vi "Delete Thing Shadow.vi"(8 "error in (no error)":errorcluster, 11 "Thing Shadow":refnum<class "Thing Shadow.lvclass">) -> (0 "error out":errorcluster)   [LabVIEW 2015, in "NI_AWS_IoT.lvlib" / "Thing Shadow.lvclass"]
uses:
  Thing Shadow.lvclass
  Core/HTTP Request/Request Options.ctl
  Core/HTTP Request/Name Value Pair.ctl
  Core/HTTP Request/Region handling.ctl
  Core/HTTP Request/URL formatting.ctl
  Thing Shadow.lvclass/Thing Shadow.ctl
  Read Thing Name.vi
  Core/HTTP Request/HTTP Request.lvclass
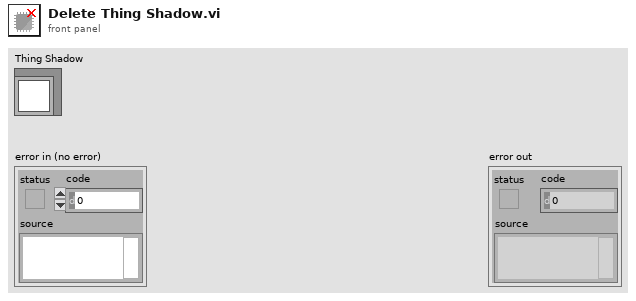
[diagram p1: front panel]
types:
  T1 = typedef "NI_AWS_Core.lvlib/HTTP Request.lvclass/Name Value Pair.ctl" = cluster{"name":string, "value":string}
  T2 = typedef "NI_AWS_Core.lvlib/HTTP Request.lvclass/Request Options.ctl" = cluster{"request headers":T1[], "request parameters":T1[], "request body":string, "region handling":T3, "URL formatting":T4}
  T3 = typedef "NI_AWS_Core.lvlib/HTTP Request.lvclass/Region handling.ctl" = enum16{"use region everywhere", "use region (authentication only)", "use region (URL only)", "ignore region everwhere"}
  T4 = typedef "NI_AWS_Core.lvlib/HTTP Request.lvclass/URL formatting.ctl" = enum16{"region-", "region."}
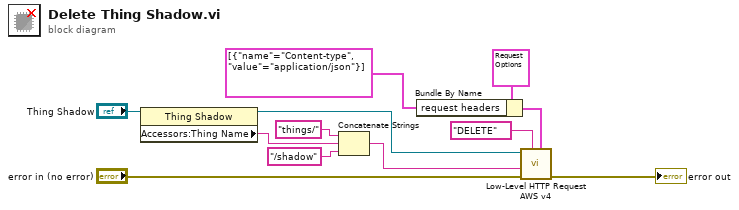
[diagram p0: block diagram]
diagram:
  n1 = property class="Thing Shadow"(reference="Thing Shadow") -> (reference out=w3:refnum<class "Thing Shadow.lvclass">, "Accessors:Thing Name"=w2:string)  [unwired: 1 in, 1 out]
  n2 = Concatenate Strings("things/" ("string"), w2, "/shadow" ("string")) -> (w7:string)
  n3 = Bundle By Name(cluster=T2 {"request headers"=[], "request parameters"=[], "request body"="", "region handling"=enum."use region everywhere", "URL formatting"=enum."region."} ("Request Options"), "request headers"=T1[] [{"name"="Content-type", "value"="application/json"}]) -> (w8:T2)
  n4 = call "Low-Level HTTP Request AWS v4.vi"("Request Options"=w8, "HTTP-Verb"="DELETE", "error in (no error)"="error in (no error)", "URL Suffix"=w7, "AWS Core in"=w3) -> ("error out"=→"error out":errorcluster)  [unwired: 3 in, 3 out]
